vi "GPS -Evnt Mouse Move.vi"(4 "User Parameter":refnum<vi>[](array[refnum]), 5 "Event Data":cluster{"sender":refnum<k24>, "e":refnum<k24>}, 6 "Control Ref":refnum<k24>, 7 "Event Common Data":T1) -> ()   [LabVIEW 2019]
uses:
  \\mac\Dropbox/gmap.net/GMAP.NET 8.6/data/GMap.NET.WindowsForms.dll
  data/GMap.NET.WindowsForms.dll
  System.Windows.Forms
  \\mac\Dropbox/gmap.net/GMAP.NET 8.6/data/GMap.NET.Core.dll
  data/GMap.NET.Core.dll
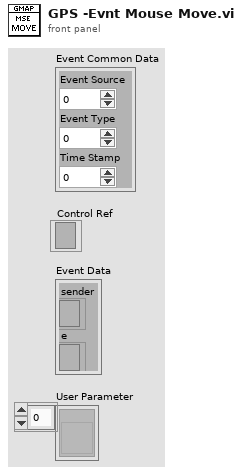
[diagram p1: front panel]
types:
  T1 = cluster{"Event Source":i32, "Event Type":u32, "Time Stamp":u32}
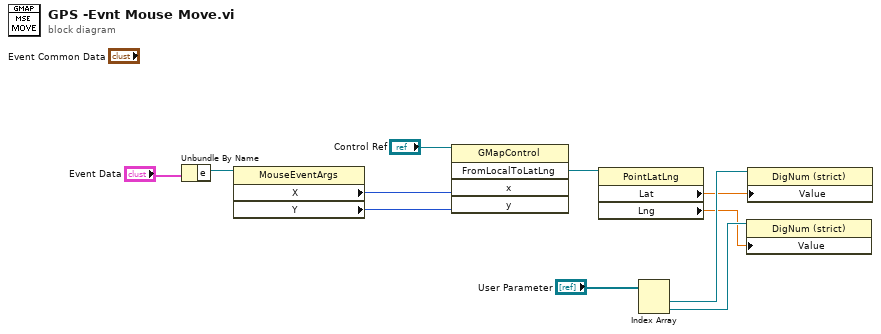
[diagram p0: block diagram]
diagram:
  n1 = Unbundle By Name("Event Data") -> ("e"=w2:refnum<k24>)
  n2 = property class="MouseEventArgs"(reference=w2) -> ("X"=w10:i32, "Y"=w9:i32)  [unwired: 1 in, 2 out]
  n3 = invoke class="GMapControl" method="FromLocalToLatLng"(reference="Control Ref", "x"=w10, "y"=w9) -> ("FromLocalToLatLng"=w11:refnum<k24>)  [unwired: 2 in, 4 out]
  n4 = property class="PointLatLng"(reference=w11) -> ("Lat"=w7:dbl, "Lng"=w5:dbl)  [unwired: 1 in, 2 out]
  n5 = Index Array(array="User Parameter") -> (element #1=w8:refnum<vi>, element #2=w6:refnum<vi>)  [unwired: 2 in]
  n6 = property class="DigNum (strict)"(reference=w6, "Value"=w5) -> ()  [unwired: 1 in, 2 out]
  n7 = property class="DigNum (strict)"(reference=w8, "Value"=w7) -> ()  [unwired: 1 in, 2 out]
